vi "ATDome_logEvent_settingsAppliedDomeTcp.vi"(8 "error in (no error)":errorcluster, 11 "logevent_settingsAppliedDomeTcp_Ctl":T1) -> (0 "error out":errorcluster, 2 "function return":i32, 3 "logevent_settingsAppliedDomeTcp_Ctl out":T1)   [LabVIEW 2016, in "SALLV_ATDome.lvlib"]
doc: "int ATDome_shm_logEvent_settingsAppliedDomeTcpLV(ATDome_logevent_settingsAppliedDomeTcpLV *logevent_settingsAppliedDomeTcp_Ctl );"
uses:
  SALLV_ATDome.lvlib
  DataTypes/logevent_settingsAppliedDomeTcp.ctl
  SALLV_ATDome.so
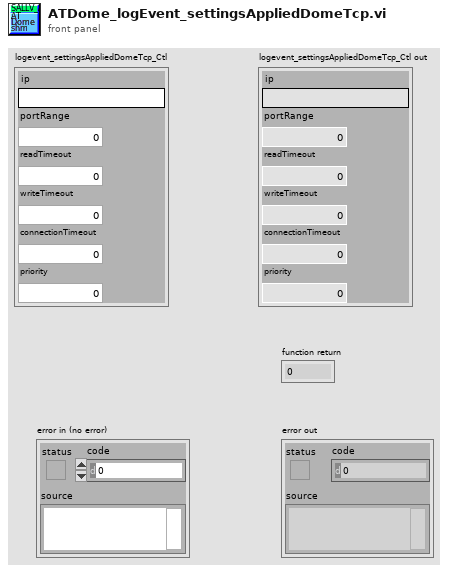
[diagram p1: front panel]
types:
  T1 = typedef "SALLV_ATDome.lvlib/logevent_settingsAppliedDomeTcp.ctl" = cluster{"ip":string, "portRange":i32, "readTimeout":sgl, "writeTimeout":sgl, "connectionTimeout":sgl, "priority":i32}
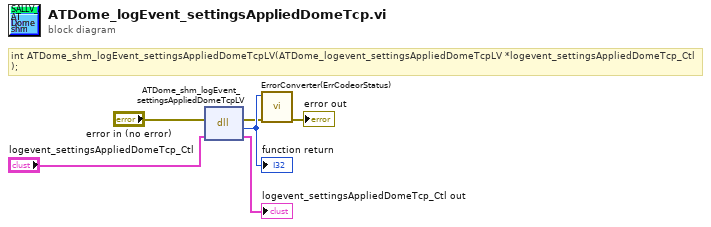
[diagram p0: block diagram]
diagram:
  # "int ATDome_shm_logEvent_settingsAppliedDomeTcpLV(ATDome_logevent_settingsAppliedDomeTcpLV *logevent_settingsAppliedDomeTcp_Ctl );"
  n1 = dll-call lib="home/andres/Desktop/SAL_ATDome/SALLV_ATDome.*" fn="ATDome_shm_logEvent_settingsAppliedDomeTcpLV"(error in="error in (no error)", "logevent_settingsAppliedDomeTcp_Ctl"="logevent_settingsAppliedDomeTcp_Ctl") -> (error out=w2:errorcluster, w6:i32, "logevent_settingsAppliedDomeTcp_Ctl"=→"logevent_settingsAppliedDomeTcp_Ctl out":T1)  [unwired: 2 in, 1 out]
  "function return" <- w6
  n2 = call "ErrorConverter(ErrCodeorStatus).vi"("error in (no error)"=w2, "error code"=w6) -> ("error out"=→"error out":errorcluster)  [unwired: 9 in]
